vi "RN SubVI.vi"() -> (4 "Numeric":i32, 6 "number: 0 to 1":dbl)   [LabVIEW 2015]
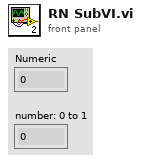
[diagram p1: front panel]
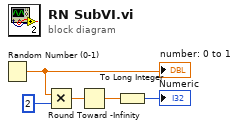
[diagram p0: block diagram]
diagram:
  n1 = Random Number (0-1)() -> (number: 0 to 1=w3:dbl)
  "number: 0 to 1" <- w3
  n2 = Multiply(x=w3, y=2) -> (x*y=w1:dbl)
  n3 = Round Toward -Infinity(1:w1) -> (0:w2:dbl)
  n4 = To Long Integer(number=w2) -> (32bit integer=→"Numeric":i32)
